vi "Extract Peaks data.vi"(1 "PMTs to monitor:":T2={"PMT 1"=TRUE, "PMT 2"=TRUE, "PMT 3"=TRUE, "PMT 4"=TRUE}, 7 "data M1,M2,M3,M4,S1,S2,S3,S4,Tin,Tout,FP":cluster{"initialized array":dbl[][]}[](array[cluster]), 12 "Acquisition rate [Hz]":dbl=100000.0 min=1.0 max=200000.0 step=1.0 format="%#_6p") -> (8 "peaks data":T1)   [LabVIEW 2009]
panel:
  out "subarray 2":dbl[](array[numeric])
  out "subarray":dbl[](array[numeric])
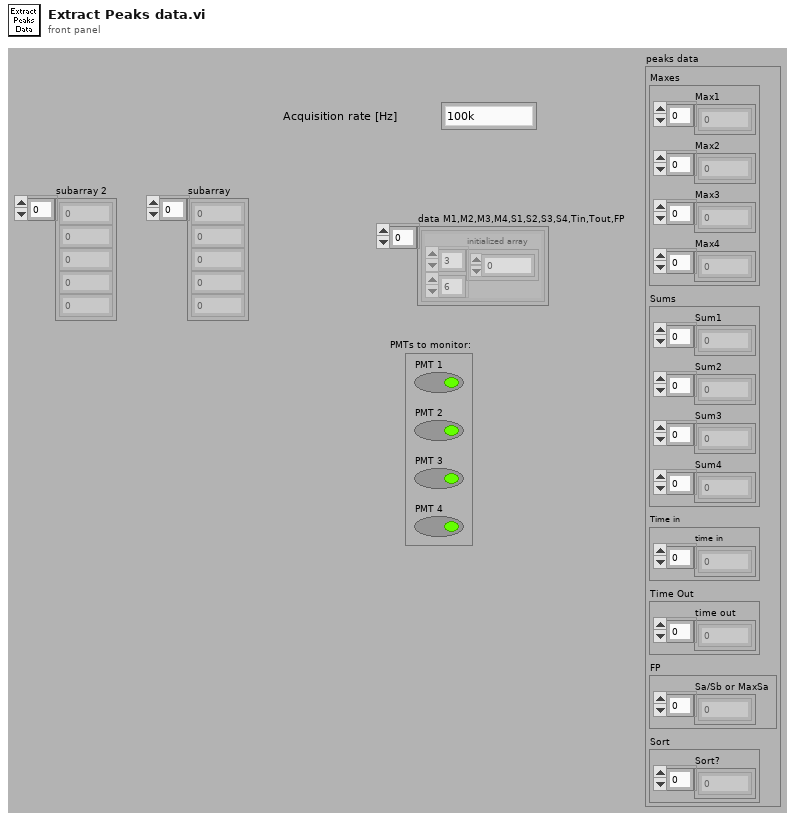
[diagram p1: front panel]
types:
  T1 = cluster{"Maxes":cluster{"Max1":dbl[], "Max2":dbl[], "Max3":dbl[], "Max4":dbl[]}, "Sums":cluster{"Sum1":dbl[], "Sum2":dbl[], "Sum3":dbl[], "Sum4":dbl[]}, "Time in":cluster{"time in":dbl[]}, "Time Out":cluster{"time out":dbl[]}, "FP":cluster{"Sa/Sb or MaxSa":dbl[]}, "Sort":cluster{"Sort?":dbl[]}}
  T2 = cluster{"PMT 1":bool, "PMT 2":bool, "PMT 3":bool, "PMT 4":bool}
  T3 = cluster{"Maxes":cluster{"Max1":dbl[], "Max2":dbl[], "Max3":dbl[], "Max4":dbl[]}, "Sums":cluster{"Sum1":dbl[], "Sum2":dbl[], "Sum3":dbl[], "Sum4":dbl[]}, "Time in":cluster{"time in":dbl[]}, "Time Out":cluster{"time out":dbl[]}, "FP":cluster{"Sa/Sb or MaxSa":dbl[]}, "Cluster 2":cluster{"Sort?":dbl[]}}
  T4 = cluster{"Max1":dbl[], "Max2":dbl[], "Max3":dbl[], "Max4":dbl[]}
  T5 = cluster{"Sum1":dbl[], "Sum2":dbl[], "Sum3":dbl[], "Sum4":dbl[]}
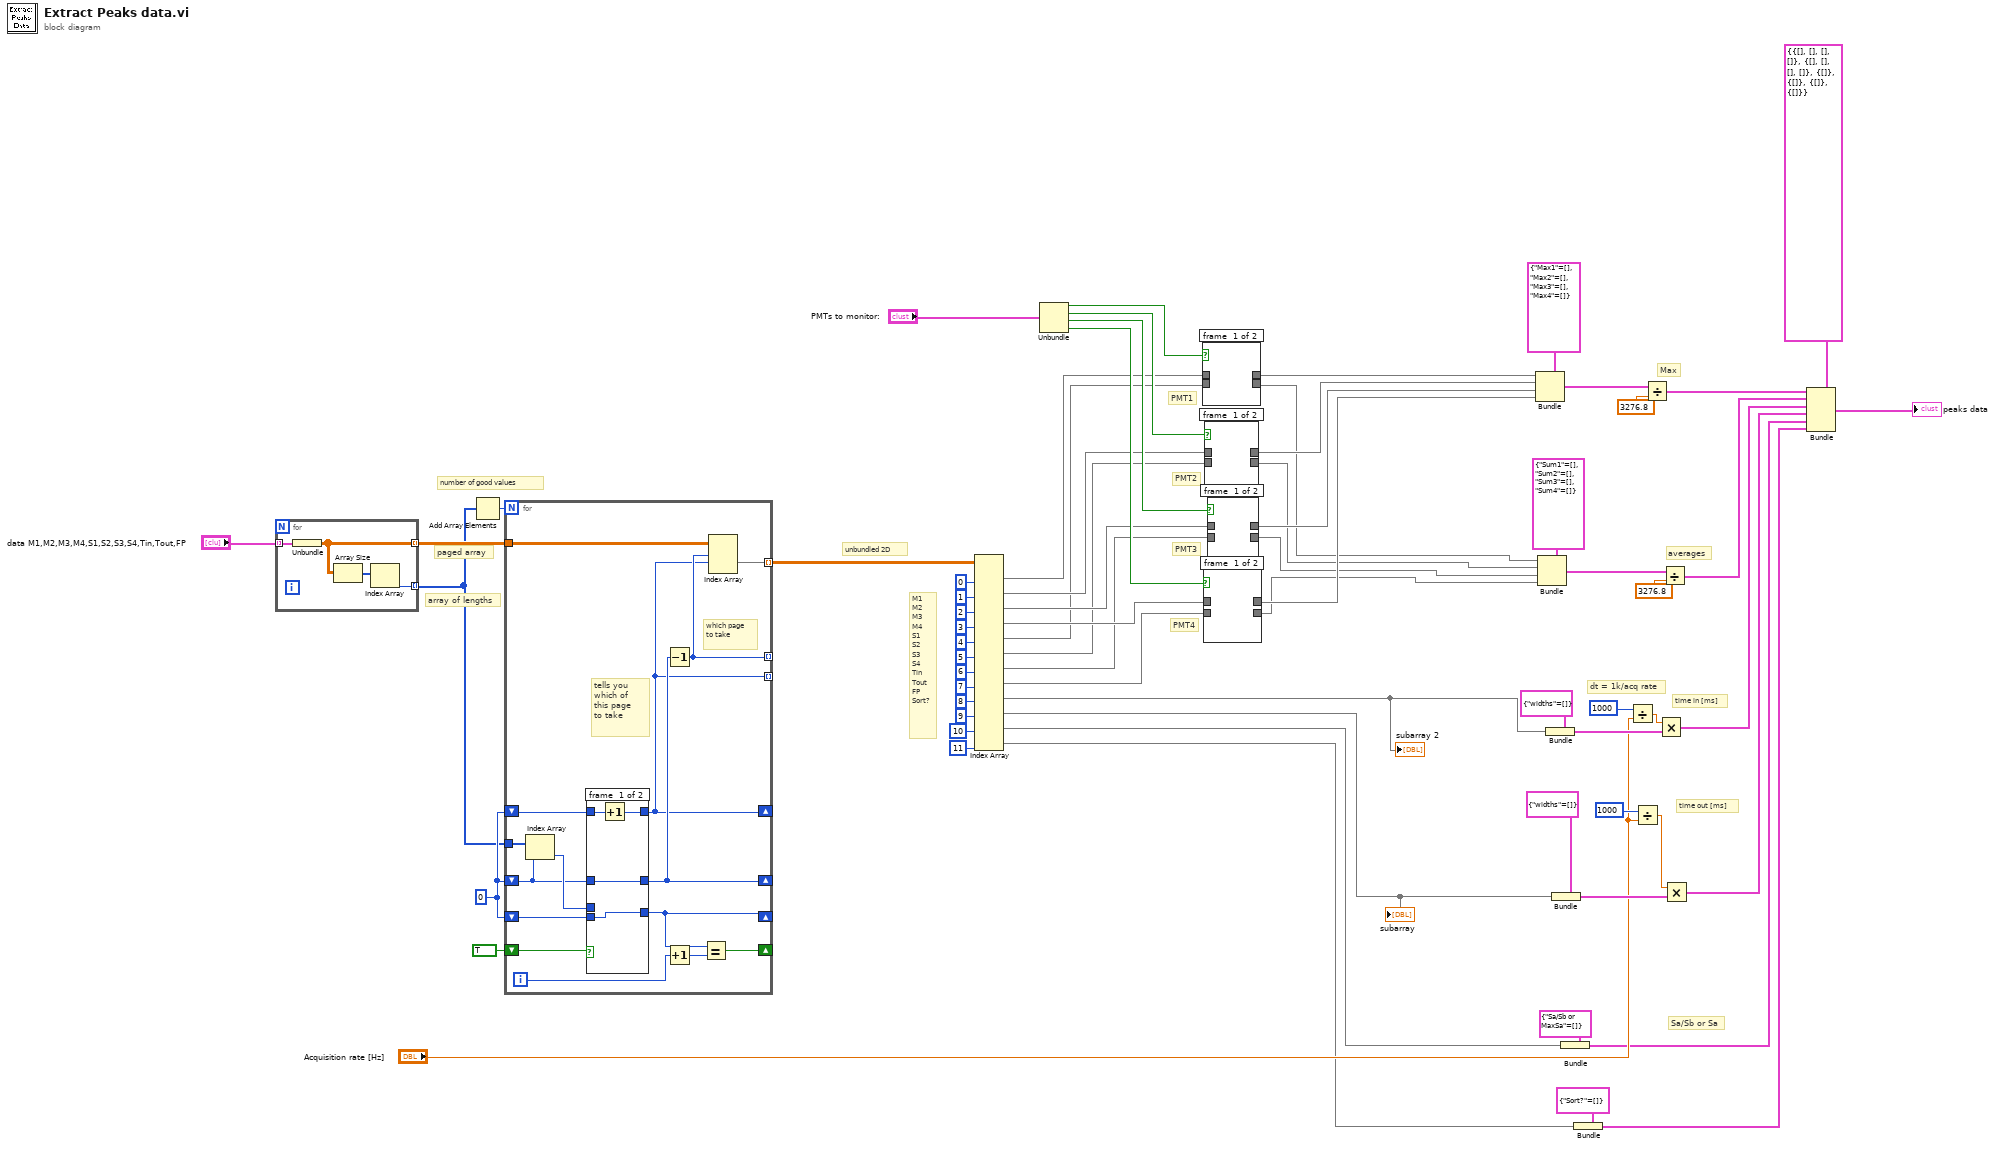
[diagram p0: block diagram]
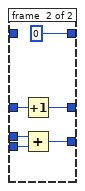
[diagram p2: hidden frame]
diagram:
  w13 = 0 ("sum")
  # "unbundled 2D"
  # "number of good values"
  # "array of lengths"
  # "paged array"
  # "time out [ms]"
  # "M1\nM2\nM3\nM4\nS1\nS2\nS3\nS4\nTin\nTout\nFP\nSort?"
  # "dt = 1k/acq rate"
  # "PMT4"
  # "PMT3"
  # "PMT2"
  # "PMT1"
  # "averages"
  # "Max"
  # "Sa/Sb or Sa"
  # "time in [ms]"
  n1 = for {
    tunnel: "data M1,M2,M3,M4,S1,S2,S3,S4,Tin,Tout,FP" -> [w73] mode=indexing
    tunnel: [w72] -> w12 mode=indexing
    tunnel: [w70] -> w11 mode=indexing
    n2 = Unbundle(w73) -> ("initialized array"=w72:dbl[][])
    n3 = Array Size(array=w72) -> (size(s)=w71:i32[])
    n4 = Index Array(array=w71) -> (element=w70:i32)  [unwired: 1 in]
  }
  n5 = Add Array Elements(numeric array=w11) -> (sum=w15:i32)
  n6 = for {
    N: w15 -> [_]
    tunnel: w11 -> [w87]
    shift-right: [w85] -> _
    shift-left: w13 -> [w88]
    shift-right: [w83] -> _
    shift-left: TRUE -> [w82]
    shift-right: [w78] -> _
    shift-left: w13 -> [w79]
    shift-right: [w75] -> _
    shift-left: w13 -> [w80]
    tunnel: [w76] -> _ mode=indexing
    tunnel: [w75] -> _ mode=indexing
    tunnel: w12 -> [w77]
    tunnel: [w74] -> w10 mode=indexing
    i -> [w84]
    # "which page to take"
    # "tells you which of this page to take"
    n7 = Index Array(array=w87, index=w79) -> (element=w86:i32)
    n8 = case shown="True" w82 {
      tunnel: w88 -> [w92 w98]
      tunnel: w86 -> [_ w97]
      tunnel: [w92 w96] -> w85
      tunnel: w79 -> [w91 w95]
      tunnel: [w91 w94] -> w78
      tunnel: [w90 0 ("sum")] -> w75
      tunnel: w80 -> [w89 _]
      frame #0 {
        n9 = Increment(x=w89) -> (x+1=w90:i32)
      }
      frame #1 {
        n10 = Increment(x=w95) -> (x+1=w94:i32)
        n11 = Add(x=w97, y=w98) -> (x+y=w96:i32)
      }
    }
    n12 = Decrement(x=w78) -> (x-1=w76:i32)
    n13 = Increment(x=w84) -> (x+1=w81:i32)
    n14 = Equal?(x=w85, y=w81) -> (x = y?=w83:bool)
    n15 = Index Array(array=w77, index (dim 0)=w76, index (dim 1)=w75) -> (element=w74:dbl[])  [unwired: 1 in]
  }
  n16 = Index Array(array=w10, index (col) #1=0 ("disabled index (col)"), index (col) #2=1 ("index (col)"), index (col) #3=2 ("index (col)"), index (col) #4=3 ("index (col)"), index (col) #5=4 ("index (col)"), index (col) #6=5 ("index (col)"), index (col) #7=6 ("index (col)"), index (col) #8=7 ("index (col)"), index (col) #9=8 ("index (col)"), index (col) #10=9 ("index (col)"), index (col) #11=10 ("index (col)"), index (col) #12=11 ("index (col)")) -> (element #1=w26:dbl[], element #2=w25:dbl[], element #3=w24:dbl[], element #4=w23:dbl[], element #5=w22:dbl[], element #6=w21:dbl[], element #7=w20:dbl[], element #8=w19:dbl[], element #9=w5:dbl[], element #10=w18:dbl[], element #11=w17:dbl[], element #12=w7:dbl[])  [unwired: 12 in]
  "subarray" <- w18
  "subarray 2" <- w5
  n17 = Unbundle("PMTs to monitor:") -> ("PMT 1"=w63:bool, "PMT 2"=w62:bool, "PMT 3"=w54:bool, "PMT 4"=w53:bool)
  n18 = case shown="True" w63 {
    tunnel: w26 -> [_ w100]
    tunnel: w22 -> [_ w99]
    tunnel: [_ w100] -> w52
    tunnel: [_ w99] -> w1
    frame #0 {
    }
    frame #1 {
    }
  }
  n19 = case shown="True" w53 {
    tunnel: w23 -> [_ w102]
    tunnel: w19 -> [_ w101]
    tunnel: [_ w102] -> w49
    tunnel: [_ w101] -> w4
    frame #0 {
    }
    frame #1 {
    }
  }
  n20 = case shown="True" w62 {
    tunnel: w25 -> [_ w104]
    tunnel: w21 -> [_ w103]
    tunnel: [_ w104] -> w51
    tunnel: [_ w103] -> w2
    frame #0 {
    }
    frame #1 {
    }
  }
  n21 = case shown="True" w54 {
    tunnel: w24 -> [_ w106]
    tunnel: w20 -> [_ w105]
    tunnel: [_ w106] -> w50
    tunnel: [_ w105] -> w3
    frame #0 {
    }
    frame #1 {
    }
  }
  n22 = Bundle(cluster=T4 {"Max1"=[], "Max2"=[], "Max3"=[], "Max4"=[]}, "Max1"=w52, "Max2"=w51, "Max3"=w50, "Max4"=w49) -> (w60:T4)
  n23 = Bundle(cluster=T5 {"Sum1"=[], "Sum2"=[], "Sum3"=[], "Sum4"=[]}, "Sum1"=w1, "Sum2"=w2, "Sum3"=w3, "Sum4"=w4) -> (w58:T5)
  n24 = Bundle(cluster=cluster{"widths":dbl[]} {"widths"=[]}, "widths"=w5) -> (w55:cluster{"widths":dbl[]})
  n25 = Bundle(cluster=cluster{"widths":dbl[]} {"widths"=[]}, "widths"=w18) -> (w48:cluster{"widths":dbl[]})
  n26 = Bundle(cluster=cluster{"Sa/Sb or MaxSa":dbl[]} {"Sa/Sb or MaxSa"=[]} ("Cluster 2"), "Sa/Sb or MaxSa"=w17) -> (w39:cluster{"Sa/Sb or MaxSa":dbl[]})
  n27 = Bundle(cluster=cluster{"Sort?":dbl[]} {"Sort?"=[]} ("Cluster 2"), "Sort?"=w7) -> (w6:cluster{"Sort?":dbl[]})
  n28 = Divide(x=1000, y="Acquisition rate [Hz]") -> (x/y=w56:dbl)
  n29 = Divide(x=1000, y="Acquisition rate [Hz]") -> (x/y=w47:dbl)
  n30 = Divide(x=w60, y=3276.8) -> (x/y=w43:T4)
  n31 = Multiply(x=w56, y=w55) -> (x*y=w41:cluster{"widths":dbl[]})
  n32 = Divide(x=w58, y=3276.8) -> (x/y=w42:T5)
  n33 = Multiply(x=w47, y=w48) -> (x*y=w40:cluster{"widths":dbl[]})
  n34 = Bundle(cluster=T3 {"Maxes"={"Max1"=[], "Max2"=[], "Max3"=[], "Max4"=[]}, "Sums"={"Sum1"=[], "Sum2"=[], "Sum3"=[], "Sum4"=[]}, "Time in"={"time in"=[]}, "Time Out"={"time out"=[]}, "FP"={"Sa/Sb or MaxSa"=[]}, "Cluster 2"={"Sort?"=[]}} ("Cluster"), "Maxes"=w43, "Sums"=w42, "Time in"=w41, "Time Out"=w40, "FP"=w39, "Cluster 2"=w6) -> (→"peaks data":T3)
